vi "To Variant.vi"(0 "Obj in":refnum<class "FSM.Port.lvclass">, 11 "error in (no error)":errorcluster) -> (4 "Obj out":refnum<class "FSM.Port.lvclass">, 8 "Array":variant[](array[variant]), 15 "error out":errorcluster)   [LabVIEW 2020, in "FSM.Port.lvclass"]
uses:
  FSM.Port.lvclass
  FSM.Port.lvclass/FSM.Port.ctl
  epl-vi-lib/Koop/KObject Class/KObject.lvclass
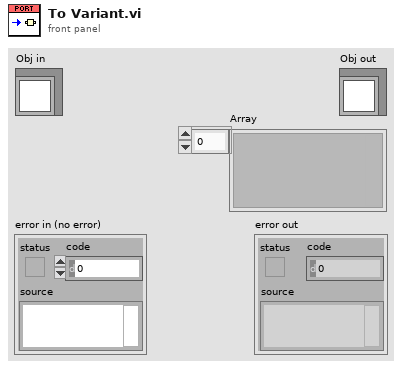
[diagram p1: front panel]
types:
  T1 = typedef "FSM.Port.lvclass/Serialized.ctl" = cluster{"Location":cluster{"x":i16, "y":i16}, "BelongsTo":string}
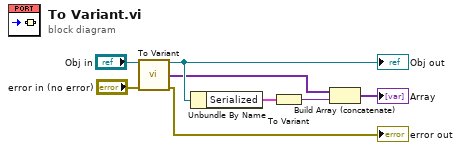
[diagram p0: block diagram]
diagram:
  n1 = call-parent "To Variant.vi"("KObject in"="Obj in", "error in (no error)"="error in (no error)") -> ("KObject out"=w3:refnum<class "FSM.Port.lvclass">, "Array"=w2:variant[], "error out"=→"error out":errorcluster)  [unwired: 11 in]
  "Obj out" <- w3
  n2 = Unbundle By Name(w3) -> ("Serialized"=w4:T1)
  n3 = To Variant(anything=w4) -> (Variant=w5:variant)
  n4 = Build Array (concatenate)(w2, w5) -> (→"Array":variant[])
